vi "WSVCAP SHL Host LL RFFE Convert Channel Bytes to Bit Array.vi"(0 "RFFE Data":u8[][](array[numeric]) format="%02x", 7 "Cycle CMD Lengths Out (bits)":u8[](array[numeric]), 9 "Cycle CMD Delay Out (ticks)":u32[](array[numeric])) -> (4 "Write Data":u64[](array[numeric]) format="%016x")   [LabVIEW 2017]
panel:
  # "D0"
  # "D4"
  # "D8"
  # "D12"
  # "D16"
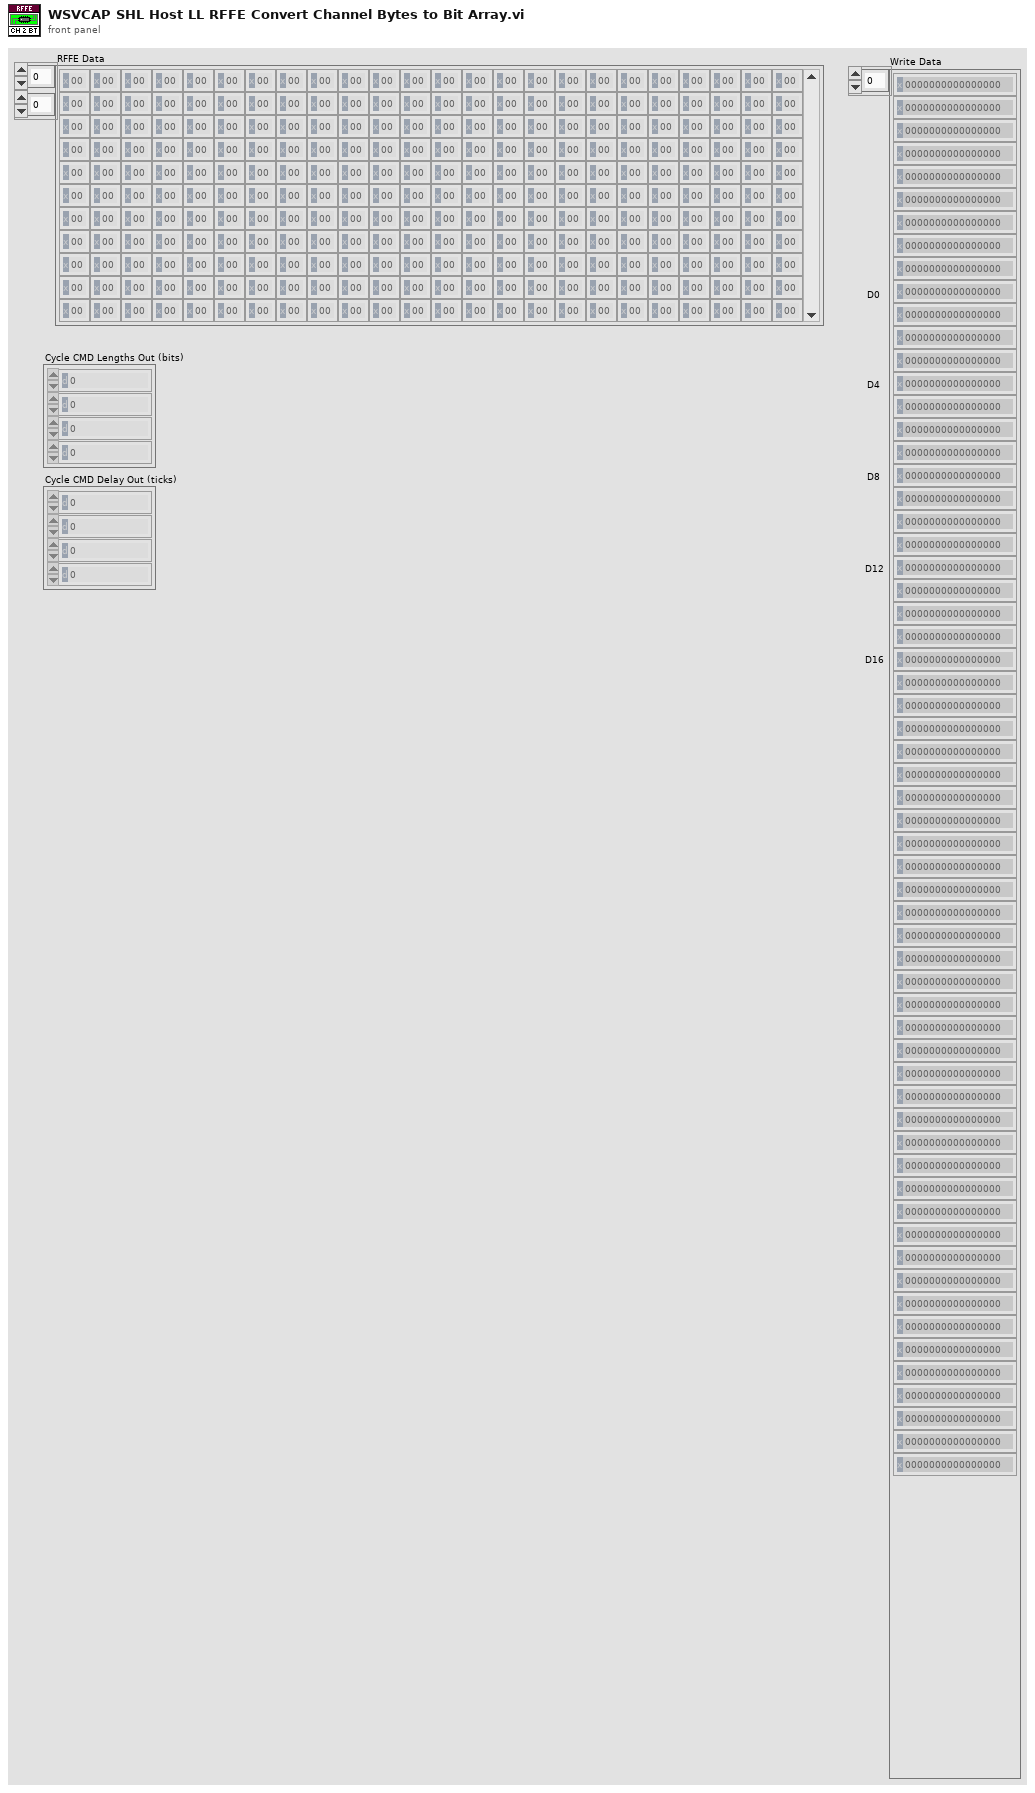
[diagram p1: front panel]
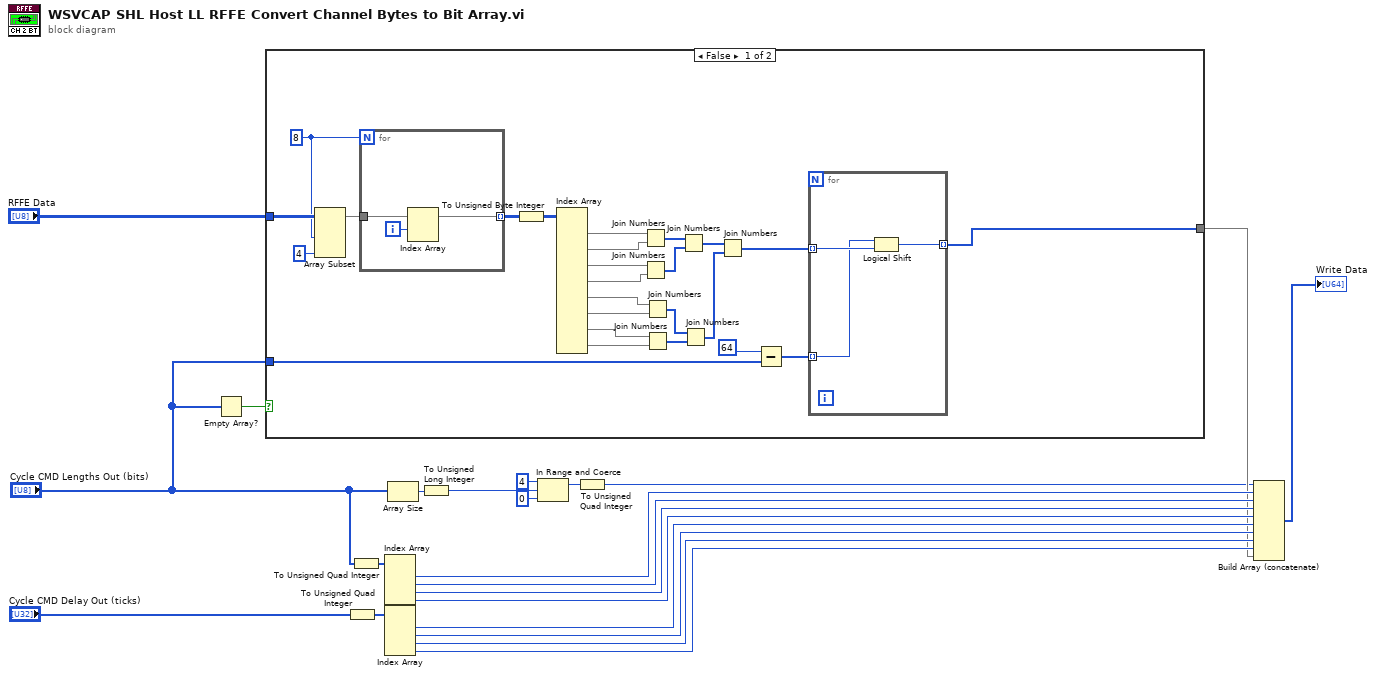
[diagram p0: block diagram]
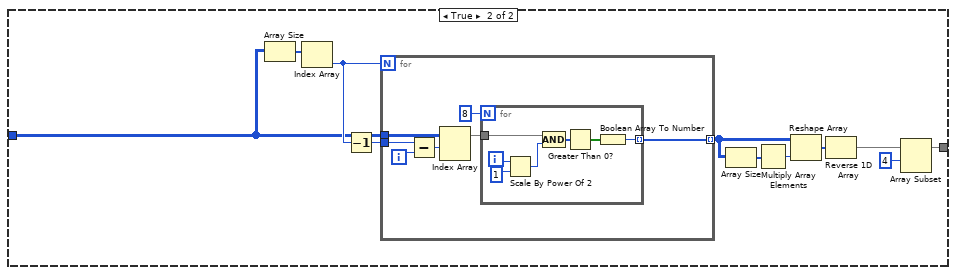
[diagram p2: hidden frame]
diagram:
  n1 = Empty Array?(array="Cycle CMD Lengths Out (bits)") -> (empty?=w4:bool)
  n2 = case shown="False" w4 {
    tunnel: "RFFE Data" -> [w35 w55]
    tunnel: [w29 w57] -> w5
    tunnel: "Cycle CMD Lengths Out (bits)" -> [w25 _]
    frame False {
      w33 = 8
      n3 = Array Subset(array=w35, length (row)=w33, length (col)=4 ("length")) -> (w34:u8[][])  [unwired: 2 in]
      n4 = for {
        N: w33 -> [_]
        tunnel: w34 -> [w53]
        tunnel: [w51] -> w36 mode=indexing
        i -> [w52]
        n5 = Index Array(array=w53, index (row)=w52) -> (element=w51:u8[])  [unwired: 1 in]
      }
      n6 = To Unsigned Byte Integer(number=w36) -> (unsigned 8bit integer=w40:u8[][])
      n7 = Index Array(array=w40) -> (element #1=w47:u8[], element #2=w46:u8[], element #3=w45:u8[], element #4=w44:u8[], element #5=w39:u8[], element #6=w31:u8[], element #7=w28:u8[], element #8=w27:u8[])  [unwired: 16 in]
      n8 = Join Numbers(hi=w47, lo=w46) -> ((hi.lo)=w43:u16[])
      n9 = Join Numbers(hi=w45, lo=w44) -> ((hi.lo)=w42:u16[])
      n10 = Join Numbers(hi=w39, lo=w31) -> ((hi.lo)=w38:u16[])
      n11 = Join Numbers(hi=w28, lo=w27) -> ((hi.lo)=w26:u16[])
      n12 = Join Numbers(hi=w43, lo=w42) -> ((hi.lo)=w41:u32[])
      n13 = Join Numbers(hi=w38, lo=w26) -> ((hi.lo)=w37:u32[])
      n14 = Join Numbers(hi=w41, lo=w37) -> ((hi.lo)=w30:u64[])
      n15 = Subtract(x=u8 64 ("length"), y=w25) -> (x-y=w23:u8[])
      n16 = for {
        tunnel: w30 -> [w50] mode=indexing
        tunnel: [w49] -> w29 mode=indexing
        tunnel: w23 -> [w48] mode=indexing
        n17 = Logical Shift(y=w48, x=w50) -> (x << y=w49:u64)
      }
    }
    frame True {
      n18 = Array Size(array=w55) -> (size(s)=w61:i32[])
      n19 = Index Array(array=w61) -> (element=w59:i32)  [unwired: 1 in]
      n20 = Decrement(x=w59) -> (x-1=w58:i32)
      n21 = for {
        N: w59 -> [_]
        tunnel: w55 -> [w69]
        tunnel: [w70] -> w64 mode=indexing
        tunnel: w58 -> [w65]
        i -> [w67]
        n22 = Subtract(x=w65, y=w67) -> (x-y=w66:i32)
        n23 = Index Array(array=w69, index (row)=w66) -> (element=w68:u8[])  [unwired: 1 in]
        n24 = for {
          N: 8 -> [_]
          tunnel: w68 -> [w74]
          tunnel: [w73] -> w70 mode=indexing
          i -> [w76]
          n25 = Scale By Power Of 2(n=w76, x=u8 1) -> (x*2^n=w77:u8)
          n26 = Compound Arithmetic op=AND(w74, w77) -> (w78:u8[])
          n27 = Greater Than 0?(x=w78) -> (x > 0?=w72:bool[])
          n28 = Boolean Array To Number(Boolean array=w72) -> (number=w73:u64)
        }
      }
      n29 = Array Size(array=w64) -> (size(s)=w63:i32[])
      n30 = Multiply Array Elements(1:w63) -> (0:w62:i32)
      n31 = Reshape Array(w64, w62) -> (w60:u64[])
      n32 = Reverse 1D Array(array=w60) -> (reversed array=w54:u64[])
      n33 = Array Subset(array=w54, index=4) -> (w57:u64[])  [unwired: 1 in]
    }
  }
  n34 = To Unsigned Quad Integer(1:"Cycle CMD Delay Out (ticks)") -> (0:w3:u64[])
  n35 = To Unsigned Quad Integer(1:"Cycle CMD Lengths Out (bits)") -> (0:w14:u64[])
  n36 = Index Array(array=w14) -> (element #1=w16:u64, element #2=w15:u64, element #3=w13:u64, element #4=w12:u64)  [unwired: 4 in]
  n37 = Index Array(array=w3) -> (element #1=w11:u64, element #2=w10:u64, element #3=w9:u64, element #4=w8:u64)  [unwired: 4 in]
  n38 = Array Size(array="Cycle CMD Lengths Out (bits)") -> (size(s)=w21:i32)
  n39 = To Unsigned Long Integer(number=w21) -> (unsigned 32bit integer=w6:u32)
  n40 = In Range and Coerce(upper limit=u32 4, x=w6, lower limit=u32 0) -> (coerced(x)=w18:u32)  [unwired: 1 out]
  n41 = To Unsigned Quad Integer(1:w18) -> (0:w2:u64)
  n42 = Build Array (concatenate)(w2, w16, w15, w13, w12, w11, w10, w9, w8, w5) -> (→"Write Data":u64[])
